vi "Configure Sequencer List All Digital Gains.vi"(7 "Digital Gains":dbl[](array[numeric]) format="%^.3e", 8 "error in (no error)":errorcluster, 10 "Instance (1)":i32=1, 11 "VISA resource name":refnum<visa-resource-name>) -> (0 "error out":errorcluster, 3 "VISA resource name out":refnum<visa-resource-name>)   [LabVIEW 2015, in "Rohde&Schwarz CMXP GPRF.lvlib"]
doc: "Defines the digital gains for all sequencer list entries.\n\nAttribute:\nRSCMXPGPRF_ATTR_SEQUENCER_LIST_ALL_DIGITAL_GAINS\n\nRemote-control command:\nSOURce:GPRF:GEN<i>:SEQuencer:LIST:DGAin:ALL"
uses:
  <instrlib>/Rohde&Schwarz CMXP GPRF/Rohde&Schwarz CMXP GPRF.lvlib
  <instrlib>/Rohde&Schwarz CMXP GPRF/Private/rsidr_core.llb/rsidr_core.lvlib
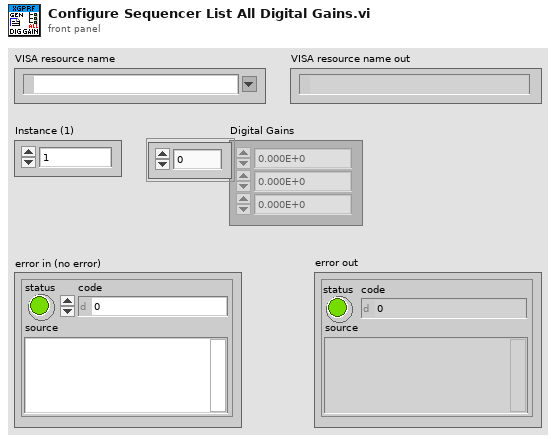
[diagram p1: front panel]
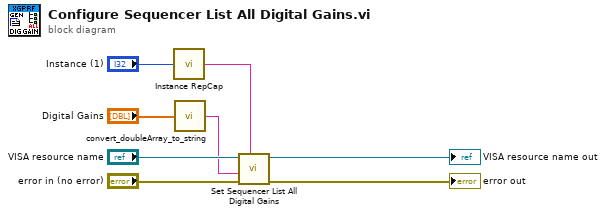
[diagram p0: block diagram]
diagram:
  n1 = call <instrlib>:"Instance RepCap.vi"("instance  in"="Instance (1)") -> ("instance out"=w8:string)
  n2 = call <instrlib>:"convert_doubleArray_to_string.vi"("double array in"="Digital Gains") -> ("string out"=w1:string)  [unwired: 4 in]
  n3 = call "Set Sequencer List All Digital Gains"("Repeated Capabilities"=w8, "error in (no error)"="error in (no error)", "Sequencer List All Digital Gains ()"=w1, "instrument handle"="VISA resource name") -> ("error out"=→"error out":errorcluster, "instrument handle out"=→"VISA resource name out":refnum<visa-resource-name>)  [unwired: 6 in]
